vi "RunDependencyInspection.vi"(8 "error in (no error)":errorcluster, 11 "CDependencyInspector in":refnum<class "CDependencyInspection.lvclass">) -> (0 "error out":errorcluster, 3 "CDependencyInspector out":refnum<class "CDependencyInspection.lvclass">)   [LabVIEW 2020, in "DependencyInspection.lvlib" / "CDependencyInspection.lvclass"]
uses:
  CDependencyInspection.lvclass
  CDependencyInspection.lvclass/CDependencyInspection.ctl
  obj/Addons/LabVIEWObjectInterfaces.lvlibp/ErrorManager/ErrorManager/ErrorType.ctl
  CRuleList/CRuleList.lvclass
  obj/Addons/LabVIEWObjectInterfaces.lvlibp/LabVIEWObjectInterfaces/ILabVIEWItem/ILabVIEWItem.lvclass
  obj/Addons/ErrorManager.lvlibp/ErrorManager/ErrorManager.lvclass
  CDependencyList/CDependencyList.lvclass
  CReporter/CReporter.lvclass
  obj/Addons/LabVIEWObjectInterfaces.lvlibp/LabVIEWObjectInterfaces/IDependencyItemRule/IDependencyItemRule.lvclass
  obj/Addons/LabVIEWObjectFactory.lvlibp
  obj/Addons/LabVIEWObjectInterfaces.lvlibp/LabVIEWObjectInterfaces/IErrorManager/IErrorManager.lvclass
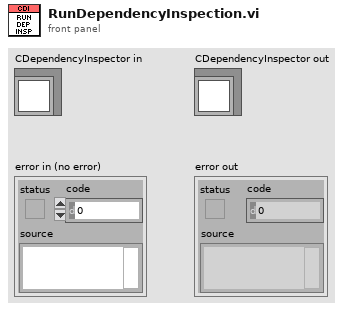
[diagram p1: front panel]
types:
  T1 = typedef "LabVIEWObjectInterfaces.lvlibp/IErrorManager.lvclass/ErrorType.ctl" = enum16{"Info", "Warning", "Error"}
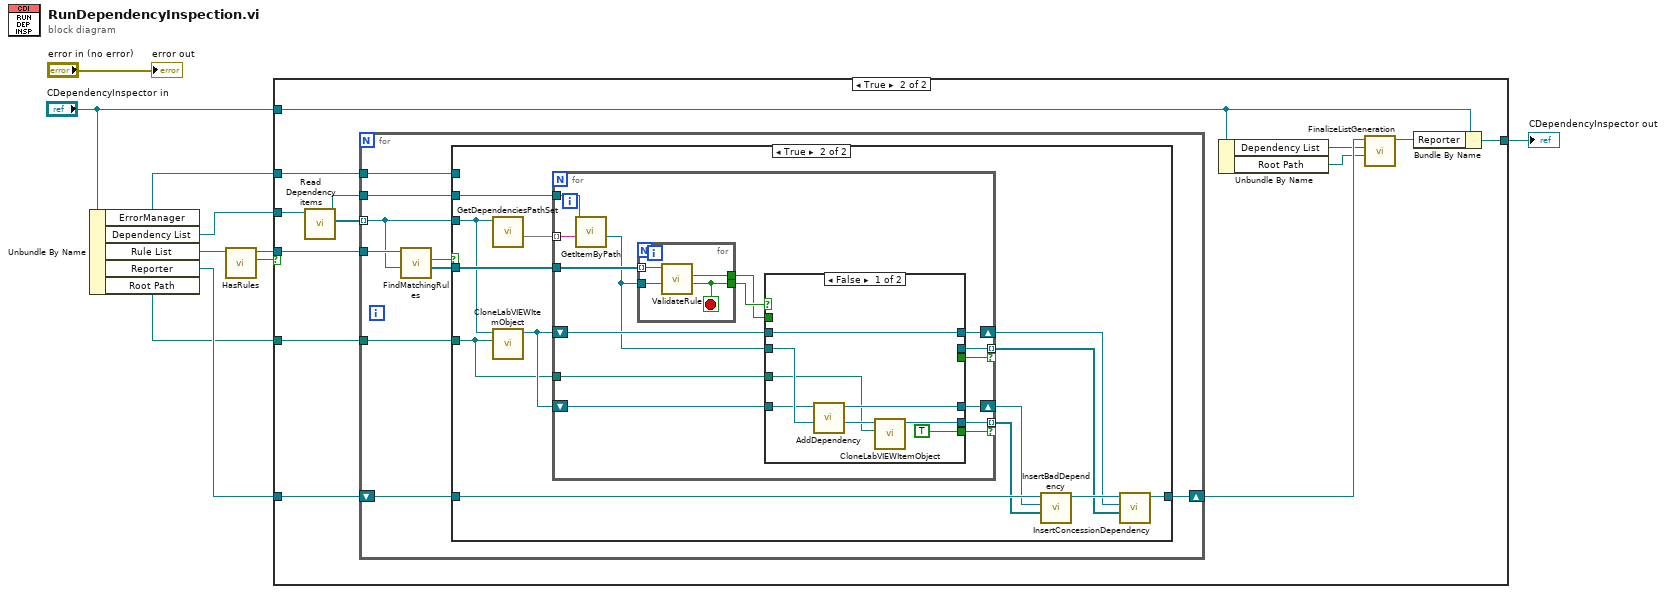
[diagram p0: block diagram]
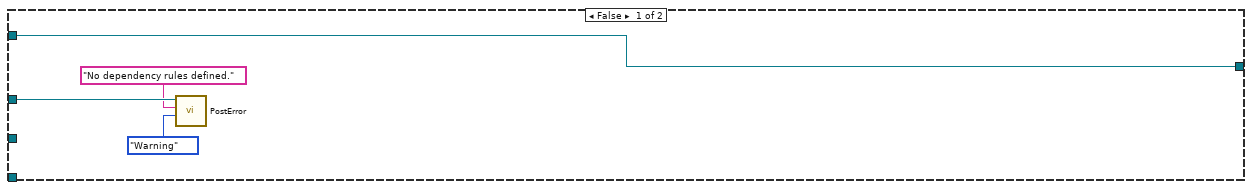
[diagram p2: hidden frame]
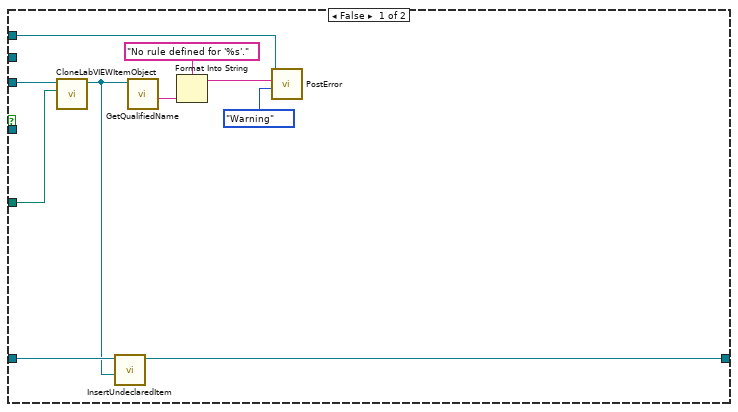
[diagram p3: hidden frame]
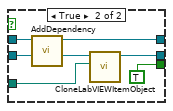
[diagram p5: hidden frame]
diagram:
  n1 = Unbundle By Name("CDependencyInspector in") -> ("ErrorManager"=w1:refnum<class "ErrorManager.lvclass">, "Dependency List"=w9:refnum<class "CDependencyList.lvclass">, "Rule List"=w4:refnum<class "CRuleList.lvclass">, "Reporter"=w8:refnum<class "CReporter.lvclass">, "Root Path"=w6:path)
  n2 = call-dynamic "HasRules.vi"("CRuleList in"=w4) -> ("Has rules?"=w2:bool, "CRuleList out"=w3:refnum<class "CRuleList.lvclass">)  [unwired: 8 in, 1 out]
  n3 = case shown="True" w2 {
    tunnel: w9 -> [_ w27]
    tunnel: w8 -> [_ w24]
    tunnel: [w14 w23] -> w7
    tunnel: w6 -> [_ w20]
    tunnel: "CDependencyInspector in" -> [w14 w19]
    tunnel: w3 -> [_ w16]
    tunnel: w1 -> [w13 w15]
    frame False {
      n4 = call-dynamic "PostError.vi"("Type"=ErrorType."Warning", "Message"="No dependency rules defined.", "ErrorManager in"=w13) -> ()  [unwired: 7 in, 2 out]
    }
    frame True {
      n5 = call-dynamic "Read Dependency items.vi"("CDependencyList in"=w27) -> ("Dependency items"=w26:refnum<class "ILabVIEWItem.lvclass">[], "CDependencyList out"=w25:refnum<class "CDependencyList.lvclass">)  [unwired: 9 in]
      n6 = for {
        tunnel: w16 -> [w35]
        tunnel: w25 -> [w36]
        tunnel: w26 -> [w34] mode=indexing
        shift-right: [w32] -> w22
        shift-left: w24 -> [w31]
        tunnel: w20 -> [w30]
        tunnel: w15 -> [w28]
        n7 = call-dynamic "FindMatchingRules.vi"("Item to match"=w34, "CRuleList in"=w35) -> ("Matching rules"=w29:refnum<class "IDependencyItemRule.lvclass">[], "rules found?"=w33:bool)  [unwired: 6 in, 2 out]
        n8 = case shown="True" w33 {
          tunnel: w36 -> [_ w52]
          tunnel: w34 -> [w46 w53]
          tunnel: w29 -> [_ w58]
          tunnel: [w44 w54] -> w32
          tunnel: w31 -> [w45 w56]
          tunnel: w30 -> [w43 w51]
          tunnel: w28 -> [w41 _]
          frame False {
            n9 = call "CloneLabVIEWItemObject.vi"("Root path"=w43, "ILabVIEWItem in"=w46) -> ("Cloned ILabVIEWItem"=w40:refnum<class "ILabVIEWItem.lvclass">)  [unwired: 9 in]
            n10 = call-dynamic "InsertUndeclaredItem.vi"("ILabVIEWItem"=w40, "CReporter in"=w45) -> ("CReporter out"=w44:refnum<class "CReporter.lvclass">)  [unwired: 8 in, 1 out]
            n11 = call-dynamic "GetQualifiedName.vi"("ILabVIEWItem in"=w40) -> ("Qualified name"=w38:string)  [unwired: 8 in, 2 out]
            n12 = Format Into String(format string="No rule defined for '%s'." ("Message"), w38) -> (resulting string=w37:string)  [unwired: 2 in, 1 out]
            n13 = call-dynamic "PostError.vi"("Type"=ErrorType."Warning", "Message"=w37, "ErrorManager in"=w41) -> ()  [unwired: 7 in, 2 out]
          }
          frame True {
            n14 = call-dynamic "GetDependenciesPathSet.vi"("ILabVIEWItem in"=w53) -> ("Dependencies"=w59:set{string})  [unwired: 8 in, 2 out]
            n15 = call "CloneLabVIEWItemObject.vi"("Root path"=w51, "ILabVIEWItem in"=w53) -> ("Cloned ILabVIEWItem"=w57:refnum<class "ILabVIEWItem.lvclass">)  [unwired: 9 in]
            n16 = for {
              tunnel: w59 -> [w73] mode=indexing
              tunnel: w52 -> [w74]
              tunnel: w58 -> [w72]
              shift-right: [w70] -> w50
              shift-left: w57 -> [w69]
              shift-right: [w68] -> w49
              shift-left: w57 -> [w67]
              tunnel: w51 -> [w64]
              tunnel: [w63] -> w48 mode=indexing if=w62
              tunnel: [w61] -> w47 mode=indexing if=w60
              n17 = call-dynamic "GetItemByPath.vi"("Path"=w73, "CDependencyList in"=w74) -> ("ILabVIEWItem"=w65:refnum<class "ILabVIEWItem.lvclass">)  [unwired: 6 in, 3 out]
              n18 = for {
                tunnel: w72 -> [w75] mode=indexing
                tunnel: w65 -> [w78]
                tunnel: [w77] -> w66
                tunnel: [w76] -> w71
                stop <- w76 stop-if-true
                n19 = call-dynamic "ValidateRule.vi"("Target"=w78, "IDependencyItemRule in"=w75) -> ("Pass?"=w76:bool, "Is concession?"=w77:bool)  [unwired: 6 in, 2 out]
              }
              n20 = case shown="False" w71 {
                tunnel: [w85 w91] -> w70
                tunnel: w69 -> [w85 w92]
                tunnel: [w82 w86] -> w68
                tunnel: w67 -> [w83 w86]
                tunnel: w66 -> [_ w93]
                tunnel: w65 -> [w84 w90]
                tunnel: w64 -> [w81 w89]
                tunnel: [w80 _] -> w63
                tunnel: [TRUE _] -> w62
                tunnel: [_ w88] -> w61
                tunnel: [_ w87] -> w60
                frame False {
                  n21 = call-dynamic "AddDependency.vi"("Item to depend on"=w84, "ILabVIEWItem in"=w83) -> ("ILabVIEWItem out"=w82:refnum<class "ILabVIEWItem.lvclass">)  [unwired: 8 in, 1 out]
                  n22 = call "CloneLabVIEWItemObject.vi"("Root path"=w81, "ILabVIEWItem in"=w84) -> ("Cloned ILabVIEWItem"=w80:refnum<class "ILabVIEWItem.lvclass">)  [unwired: 9 in]
                }
                frame True {
                  n23 = case shown="False" w93 {
                    tunnel: w92 -> [w94 w100]
                    tunnel: [w94 w98] -> w91
                    tunnel: w90 -> [_ w99]
                    tunnel: w89 -> [_ w95]
                    tunnel: [_ w97] -> w88
                    tunnel: [_ TRUE] -> w87
                    frame False {
                    }
                    frame True {
                      n24 = call-dynamic "AddDependency.vi"("Item to depend on"=w99, "ILabVIEWItem in"=w100) -> ("ILabVIEWItem out"=w98:refnum<class "ILabVIEWItem.lvclass">)  [unwired: 8 in, 1 out]
                      n25 = call "CloneLabVIEWItemObject.vi"("Root path"=w95, "ILabVIEWItem in"=w99) -> ("Cloned ILabVIEWItem"=w97:refnum<class "ILabVIEWItem.lvclass">)  [unwired: 9 in]
                    }
                  }
                }
              }
            }
            n26 = call-dynamic "InsertBadDependency.vi"("Dependency items"=w48, "ILabVIEWItem"=w49, "CReporter in"=w56) -> ("CReporter out"=w55:refnum<class "CReporter.lvclass">)  [unwired: 7 in, 1 out]
            n27 = call-dynamic "InsertConcessionDependency.vi"("Dependency items"=w47, "ILabVIEWItem"=w50, "CReporter in"=w55) -> ("CReporter out"=w54:refnum<class "CReporter.lvclass">)  [unwired: 7 in, 1 out]
          }
        }
      }
      n28 = Unbundle By Name(w19) -> ("Dependency List"=w18:refnum<class "CDependencyList.lvclass">, "Root Path"=w17:path)
      n29 = call-dynamic "FinalizeListGeneration.vi"("Root path"=w17, "CDependencyList in"=w18, "CReporter in"=w22) -> ("CReporter out"=w21:refnum<class "CReporter.lvclass">)  [unwired: 7 in, 1 out]
      n30 = Bundle By Name(cluster=w19, "Reporter"=w21) -> (w23:refnum<class "CDependencyInspection.lvclass">)
    }
  }
  "CDependencyInspector out" <- w7
  "error out" <- "error in (no error)"
